vi "ShowDialog.vi"(11 "Comm":T1) -> ()   [LabVIEW 2016]
uses:
  Errors_Global.vi
  HTTPComm.ctl
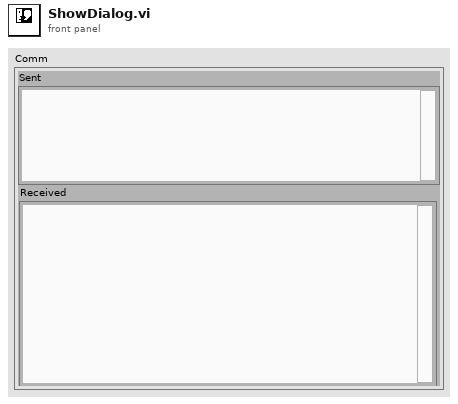
[diagram p1: front panel]
types:
  T1 = typedef "HTTPComm.ctl" = cluster{"url":string, "sent headers":string, "sent body":string, "headers":string, "body":string, "Sent":string, "Received":string}
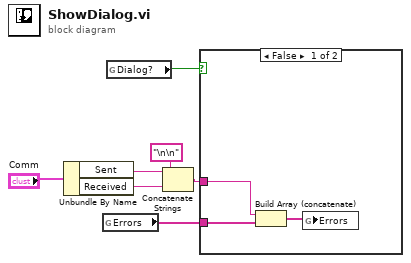
[diagram p0: block diagram]
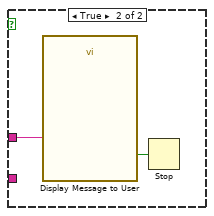
[diagram p2: hidden frame]
diagram:
  n1 = Unbundle By Name("Comm") -> ("Sent"=w6:string, "Received"=w5:string)
  n2 = global read "Errors_Global.vi" "Errors"() -> (w1:string[])
  n3 = global read "Errors_Global.vi" "Dialog?"() -> (w2:bool)
  n4 = Concatenate Strings(w6, "\n\n" ("string"), w5) -> (w4:string)
  n5 = case shown="False" w2 {
    tunnel: w4 -> [w8 w12]
    tunnel: w1 -> [w10 _]
    frame False {
      n6 = Build Array (concatenate)(w8, w10) -> (w9:string[])
      n7 = global write "Errors_Global.vi" "Errors"(w9) -> ()
    }
    frame True {
      n8 = call "Display Message to User"("Message"=w12) -> ("Abort"=w11:bool)  [unwired: 9 in, 1 out]
      n9 = Stop(stop? (T)=w11) -> ()
    }
  }
